vi "Save_Time_Traces_low.vi"(0 "Data Type":T1, 1 "Full Header Info?":bool, 2 "Put each block into separate file":bool, 3 "Precision":i16=2, 5 "No of desired samples/ch":i32, 7 "Data to save":i32[](array[ring])=[1] items=["LDA (V)", "LDA (U)", "Save Nothing"], 9 "File Extension":string=".xls", 11 "Down Sample":i32=1, 12 "Leave space between blocks?":bool, 13 "Time Series":enum16{"Milliseconds", "Seconds"}(ring), 14 "Separation Character":string="\t") -> ()   [LabVIEW 2011]
uses:
  Controls/Instrument_Array.ctl
  Globals/Meas_global.vi
  Acquisition/PWA/PWAtasksGLOBAL.vi
  Globals/Plug_in_data_global.vi
  Globals/LDA_meas_global_1.vi
panel:
  # "Run this VI to update the channel names"
  # "0 means disabled"
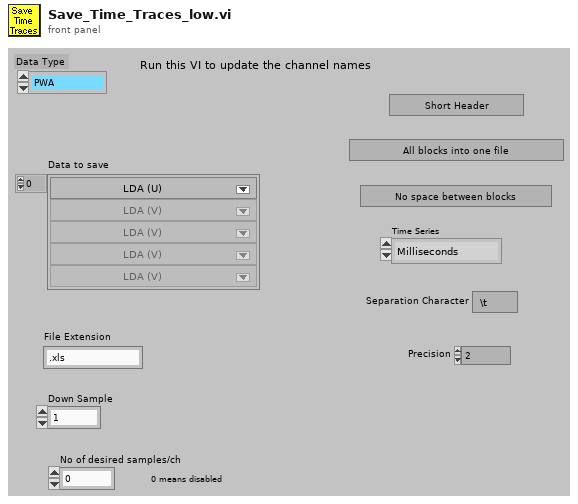
[diagram p1: front panel]
types:
  T1 = typedef "Instrument_Array.ctl" = enum16{"PWA", "LDA", "Analogue"}
  T2 = typedef "Analysis_info_cluster.ctl" = cluster{"Colour":u32, "Inst type":T3, "Inst name":string, "Symbol":string, "Code name":string, "Extra Info":string, "Inst Array":T1, "Index":i32, "Voltage Index":i32, "Extra Titles":string[], "Extra Values":string[]}
  T3 = typedef "Inst_type.ctl" = enum16{"Propeller anemometer", "Raw voltage", "Pressure Transducer", "Pitot-static tube", "Preston tube", "Hot wire", "Cross wire 1", "Cross wire 2", "Generic Linear", "Generic Polynomial", "Generic BackPoly", "Fast FID", "Thermocouple", "Cold wire", "Pulsed Wire", "LDA Vel", "LDA Tran time", "LDA Arr time"}
  T4 = typedef "Trigger_Mode.ctl" = enum16{"Free Running", "Start on Trigger", "Trigger Every Block", "Trigger Every Sample"}
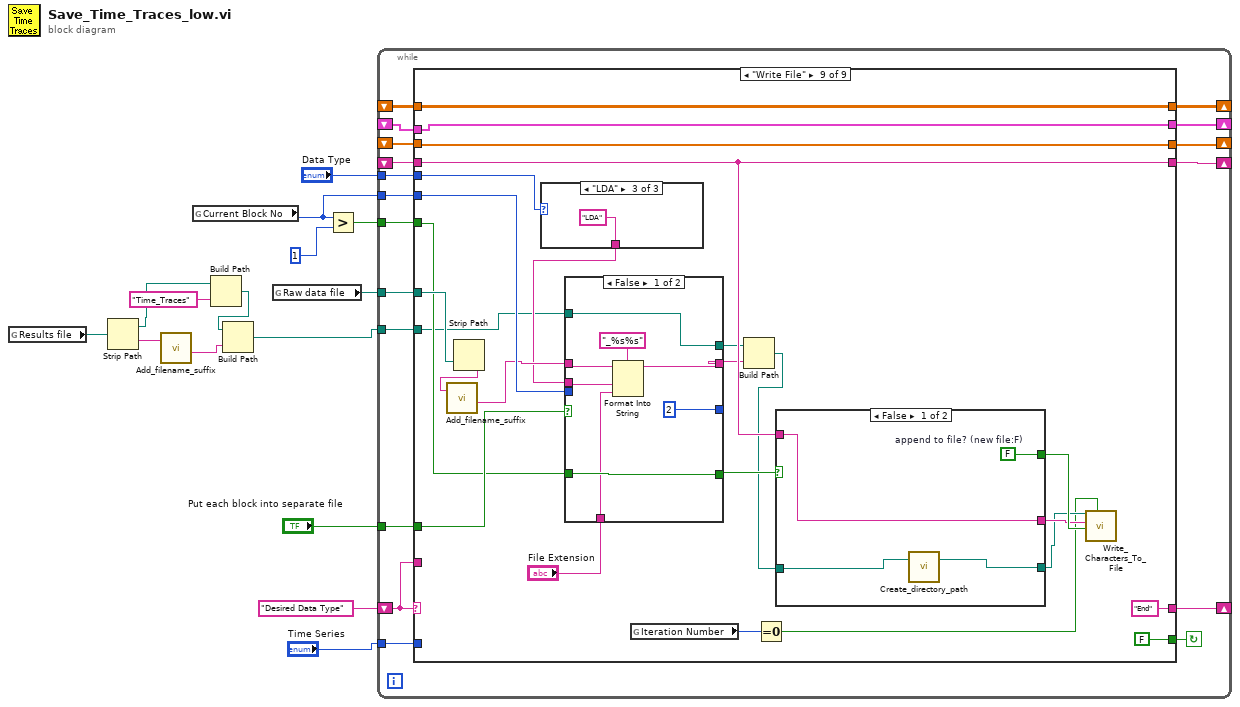
[diagram p0: block diagram]
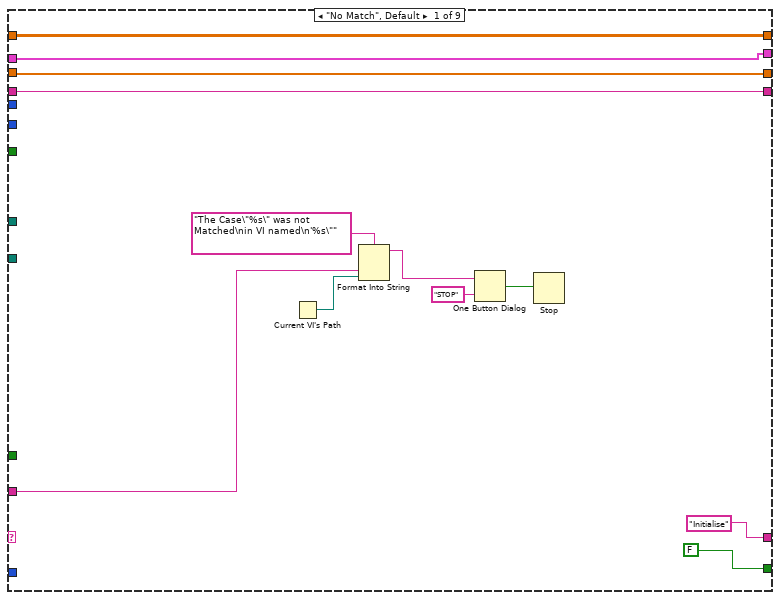
[diagram p2: hidden frame]
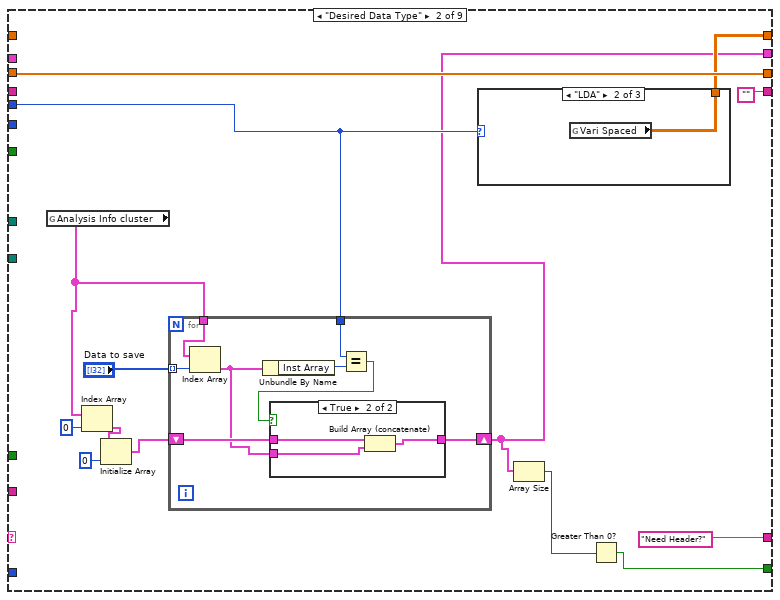
[diagram p3: hidden frame]
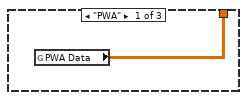
[diagram p5: hidden frame]
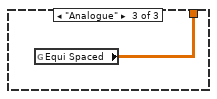
[diagram p6: hidden frame]
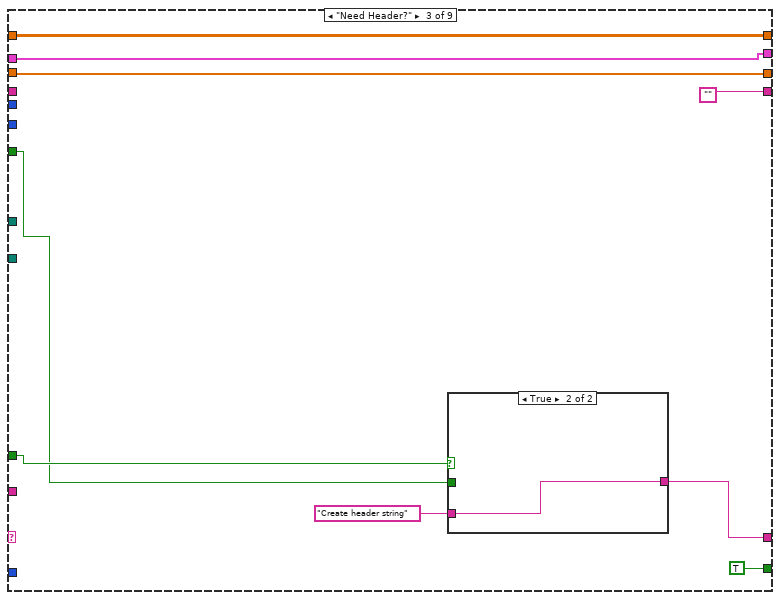
[diagram p7: hidden frame]
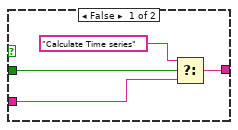
[diagram p8: hidden frame]
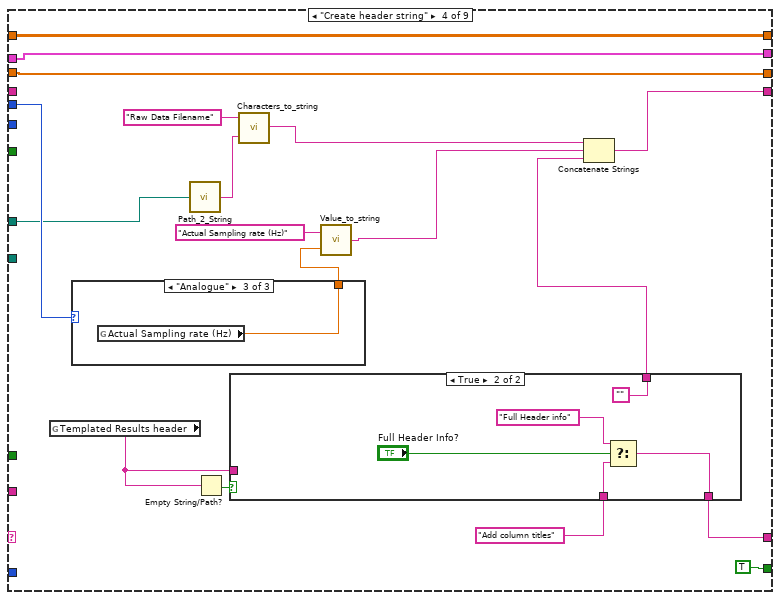
[diagram p9: hidden frame]
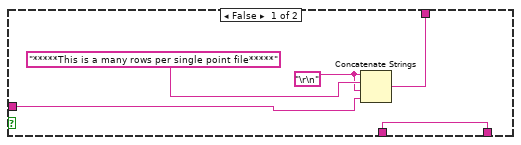
[diagram p10: hidden frame]
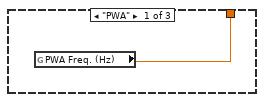
[diagram p11: hidden frame]
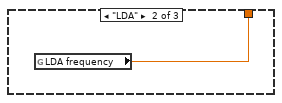
[diagram p12: hidden frame]
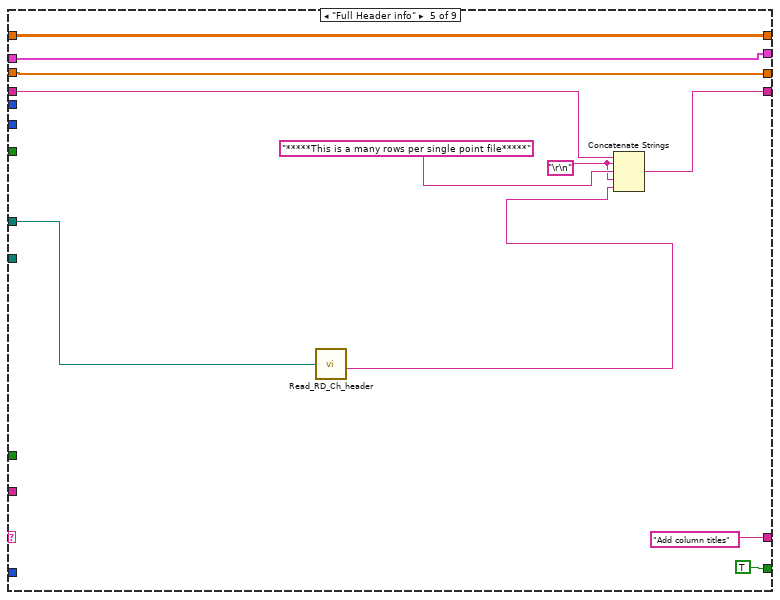
[diagram p13: hidden frame]
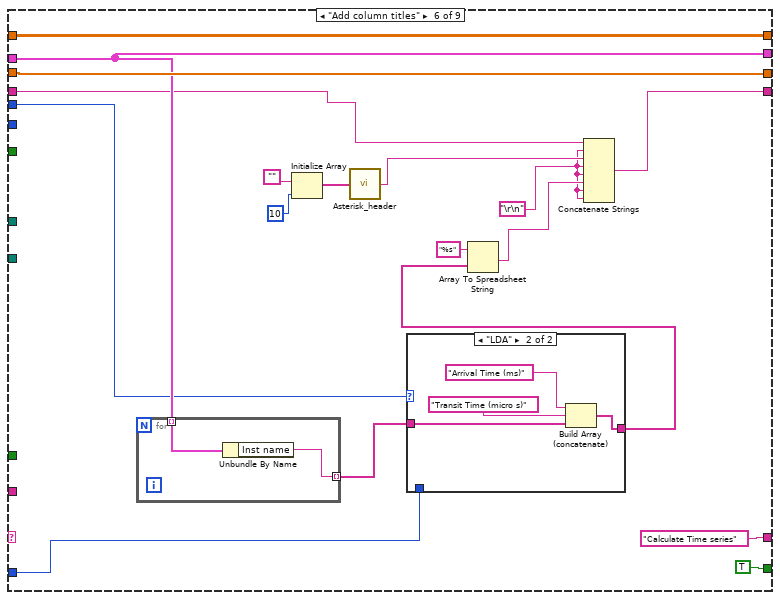
[diagram p14: hidden frame]
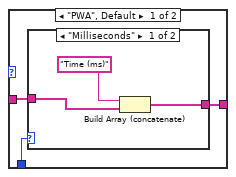
[diagram p15: hidden frame]
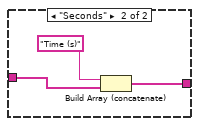
[diagram p16: hidden frame]
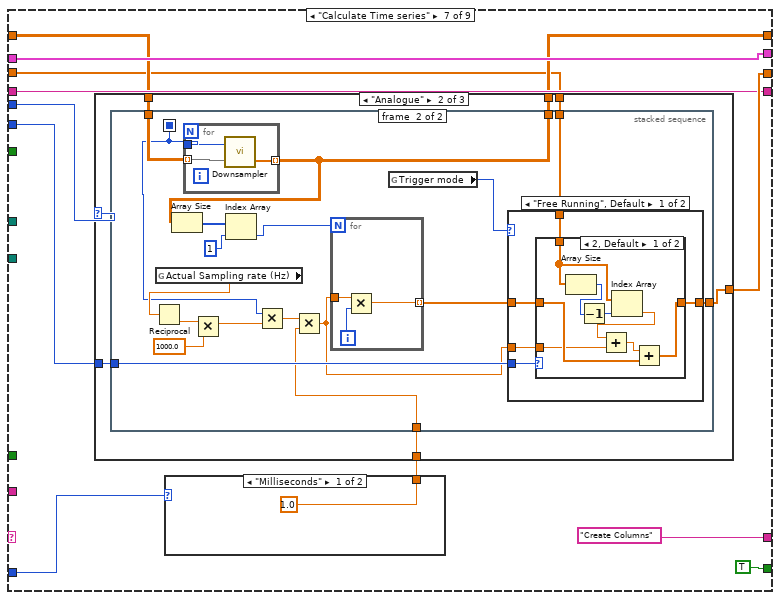
[diagram p17: hidden frame]
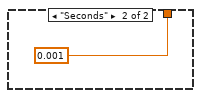
[diagram p18: hidden frame]
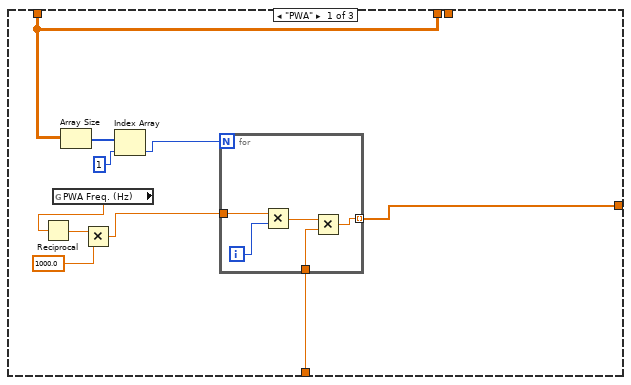
[diagram p19: hidden frame]
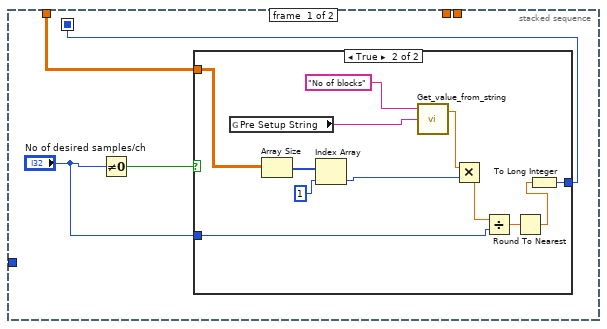
[diagram p20: hidden frame]
diagram:
  n1 = global read "Meas_global.vi" "Results file"() -> (w7:path)
  n2 = Strip Path(path=w7) -> (stripped path=w3:path, name=w6:string)
  n3 = call "Add_filename_suffix.vi"("Filename"=w6) -> ("Base name"=w5:string)  [unwired: 1 in, 3 out]
  n4 = global read "Meas_global.vi" "Current Block No"() -> (w11:i32)
  n5 = Build Path(base path=w3, name or relative path="Time_Traces") -> (appended path=w1:path)
  n6 = Build Path(base path=w1, name or relative path=w5) -> (appended path=w4:path)
  n7 = global read "Meas_global.vi" "Raw data file"() -> (w8:path)
  n8 = Greater?(x=w11, y=1) -> (0:w12:bool)
  n9 = while {
    shift-left: "Desired Data Type" -> [w31]
    shift-right: [w32] -> _
    shift-right: [w28] -> _
    shift-left: _ -> [w27]
    tunnel: "Put each block into separate file" -> [w30]
    tunnel: w8 -> [w29]
    tunnel: w12 -> [w26]
    shift-right: [w25] -> _
    shift-left: _ -> [w24]
    tunnel: w11 -> [w23]
    shift-right: [w22] -> _
    shift-left: _ -> [w21]
    tunnel: "Time Series" -> [w20]
    tunnel: "Data Type" -> [w19]
    shift-right: [w18] -> _
    shift-left: _ -> [w17]
    tunnel: w4 -> [w16]
    stop <- w33 continue-if-true
    n10 = case shown="\"Write File\"" w31 {
      tunnel: [FALSE w47 TRUE TRUE TRUE TRUE TRUE TRUE FALSE] -> w33
      tunnel: ["Initialise" "Need Header?" w80 w90 "Add column titles" ("t") "Calculate Time series" ("t") "Create Columns" ("t") "Write File" "End" ("t")] -> w32
      tunnel: w31 -> [w40 _ _ _ _ _ _ _ _]
      tunnel: w30 -> [_ _ w79 _ _ _ _ _ w346]
      tunnel: w29 -> [_ _ _ w95 w121 _ _ _ w356]
      tunnel: [w37 "" "" w103 w122 w146 w172 w273 w352] -> w28
      tunnel: w27 -> [w37 _ _ _ w123 w137 w172 w275 w352]
      tunnel: w26 -> [_ _ w78 _ _ _ _ _ w342]
      tunnel: [w36 w58 w82 w102 w129 w144 w174 w267 w349] -> w25
      tunnel: w24 -> [w36 w58 w82 w102 w129 w144 w165 w267 w349]
      tunnel: w23 -> [_ _ _ _ _ _ w164 _ w348]
      tunnel: [w35 w57 w75 w99 w128 w142 w166 w271 w343] -> w22
      tunnel: w21 -> [w35 _ w75 w99 w128 w142 w167 w271 w343]
      tunnel: w20 -> [_ _ _ _ _ w131 w171 w270 _]
      tunnel: w19 -> [_ w54 _ w97 _ w134 w169 w266 w338]
      tunnel: [w34 w46 w76 w96 w126 w141 w168 w268 w339] -> w18
      tunnel: w17 -> [w34 _ w76 w96 w126 w141 w168 w268 w339]
      tunnel: w16 -> [_ _ _ _ _ _ _ _ w335]
      frame "No Match", Default {
        n11 = Current VI's Path() -> (path=w39:path)
        n12 = Format Into String(format string="The Case\"%s\" was not Matched\nin VI named\n'%s\"" ("Format String"), w40, w39) -> (resulting string=w43:string)  [unwired: 2 in, 1 out]
        n13 = One Button Dialog(message=w43, button name ("OK")="STOP") -> (true=w41:bool)
        n14 = Stop(stop? (T)=w41) -> ()
      }
      frame "Desired Data Type" {
        n15 = global read "Meas_global.vi" "Analysis Info cluster"() -> (w50:T2[])
        n16 = Index Array(array=w50, index=0) -> (element=w51:T2)
        n17 = Initialize Array(w51, 0 ("dimension size")) -> (w53:T2[])
        n18 = for {
          tunnel: w50 -> [w67]
          tunnel: "Data to save" -> [w66] mode=indexing
          tunnel: w54 -> [w64]
          shift-right: [w60] -> w46
          shift-left: w53 -> [w62]
          n19 = Index Array(array=w67, index=w66) -> (element=w61:T2)
          n20 = Unbundle By Name(w61) -> ("Inst Array"=w65:T1)
          n21 = Equal?(x=w64, y=w65) -> (x = y?=w63:bool)
          n22 = case shown="True" w63 {
            tunnel: w62 -> [w68 w71]
            tunnel: w61 -> [_ w70]
            tunnel: [w68 w69] -> w60
            frame False {
            }
            frame True {
              n23 = Build Array (concatenate)(w71, w70) -> (w69:T2[])
            }
          }
        }
        n24 = case shown="\"LDA\"" w54 {
          tunnel: [w72 w73 w74] -> w57
          frame "PWA" {
            n25 = global read "PWAtasksGLOBAL.vi" "PWA Data"() -> (w72:dbl[][])
          }
          frame "LDA" {
            n26 = global read "Plug_in_data_global.vi" "Vari Spaced"() -> (w73:dbl[][])
          }
          frame "Analogue" {
            n27 = global read "Plug_in_data_global.vi" "Equi Spaced"() -> (w74:dbl[][])
          }
        }
        n28 = Array Size(array=w46) -> (size(s)=w48:i32)
        n29 = Greater Than 0?(x=w48) -> (x > 0?=w47:bool)
      }
      frame "Need Header?" {
        n30 = case shown="True" w79 {
          tunnel: [w87 w88] -> w80
          tunnel: w78 -> [w86 _]
          tunnel: "Create header string" -> [w84 w88]
          frame False {
            n31 = Select(t="Calculate Time series", s=w86, f=w84) -> (s? t:f=w87:string)
          }
          frame True {
          }
        }
      }
      frame "Create header string" {
        n32 = global read "Plug_in_data_global.vi" "Templated Results header"() -> (w92:string)
        n33 = case shown="\"Analogue\"" w97 {
          tunnel: [w117 w118 w119] -> w98
          frame "PWA" {
            n34 = global read "PWAtasksGLOBAL.vi" "PWA Freq. (Hz)"() -> (w117:dbl)
          }
          frame "LDA" {
            n35 = global read "Meas_global.vi" "LDA frequency"() -> (w118:dbl)
          }
          frame "Analogue" {
            n36 = global read "Meas_global.vi" "Actual Sampling rate (Hz)"() -> (w119:dbl)
          }
        }
        n37 = call "Path_2_String.vi"("Real Path"=w95) -> ("Path String"=w94:string)
        n38 = Empty String/Path?(string/path=w92) -> (empty?=w93:bool)
        n39 = case shown="True" w93 {
          tunnel: w92 -> [w109 _]
          tunnel: "Add column titles" ("t") -> [w108 w114]
          tunnel: [w108 w113] -> w90
          tunnel: [w107 ""] -> w89
          frame False {
            w110 = "\r\n"
            n40 = Concatenate Strings(w110, "*****This is a many rows per single point file*****", w110, w109) -> (w107:string)
          }
          frame True {
            n41 = Select(t="Full Header info", s="Full Header Info?", f=w114) -> (s? t:f=w113:string)
          }
        }
        n42 = call "Characters_to_string.vi"("Characters to write"=w94, "Label for characters"="Raw Data Filename") -> ("Output string"=w105:string)
        n43 = call "Value_to_string.vi"("Value"=w98, "Label for value"="Actual Sampling rate (Hz)") -> ("Output string"=w100:string)  [unwired: 1 in]
        n44 = Concatenate Strings(w105, w100, w89) -> (w103:string)
      }
      frame "Full Header info" {
        w124 = "\r\n"
        n45 = call "Read_RD_Ch_header.vi"("Raw data file"=w121) -> ("Ch string"=w120:string)  [unwired: 3 out]
        n46 = Concatenate Strings(w123, w124, "*****This is a many rows per single point file*****", w124, w120) -> (w122:string)
      }
      frame "Add column titles" {
        w135 = "\r\n"
        n47 = for {
          tunnel: [w162] -> w133 mode=indexing
          tunnel: w141 -> [w163] mode=indexing
          n48 = Unbundle By Name(w163) -> ("Inst name"=w162:string)
        }
        n49 = Initialize Array("", 10) -> (w138:string[])
        n50 = call "Asterisk_header.vi"("Channel names"=w138) -> ("Header string"=w136:string)
        n51 = case shown="\"LDA\"" w134 {
          tunnel: w133 -> [w151 w159]
          tunnel: [w150 w158] -> w132
          tunnel: w131 -> [w149 _]
          frame "PWA", Default {
            n52 = case shown="\"Milliseconds\"" w149 {
              tunnel: w151 -> [w154 w157]
              tunnel: [w153 w156] -> w150
              frame "Milliseconds" {
                n53 = Build Array (concatenate)("Time (ms)", w154) -> (w153:string[])
              }
              frame "Seconds" {
                n54 = Build Array (concatenate)("Time (s)", w157) -> (w156:string[])
              }
            }
          }
          frame "LDA" {
            n55 = Build Array (concatenate)("Arrival Time (ms)", "Transit Time (micro s)", w159) -> (w158:string[])
          }
        }
        n56 = Array To Spreadsheet String(array=w132, 3:"%s" ("format string")) -> (spreadsheet string=w143:string)  [unwired: 1 out]
        n57 = Concatenate Strings(w137, w135, w136, w135, w135, w143, w135, w135) -> (w146:string)
      }
      frame "Calculate Time series" {
        n58 = case shown="\"Milliseconds\"" w171 {
          tunnel: [1.0 0.001] -> w170
          frame "Milliseconds" {
          }
          frame "Seconds" {
          }
        }
        n59 = case shown="\"Analogue\"" w169 {
          tunnel: [w179 w195 w256] -> w174
          tunnel: w170 -> [w181 w198 w257]
          tunnel: w167 -> [w178 w197 w255]
          tunnel: [w178 w196 w255] -> w166
          tunnel: w165 -> [_ w194 _]
          tunnel: w164 -> [_ w193 _]
          frame "PWA" {
            n60 = global read "PWAtasksGLOBAL.vi" "PWA Freq. (Hz)"() -> (w180:dbl)
            n61 = Reciprocal(x=w180) -> (1/x=w187:dbl)
            n62 = Array Size(array=w178) -> (size(s)=w184:i32[])
            n63 = Multiply(x=w187, y=1000.0) -> (x*y=w185:dbl)
            n64 = Index Array(array=w184, index=1) -> (element=w182:i32)
            n65 = for {
              N: w182 -> [_]
              tunnel: w185 -> [w191]
              tunnel: [w189] -> w179 mode=indexing
              tunnel: w181 -> [w188]
              i -> [w192]
              n66 = Multiply(x=w191, y=w192) -> (x*y=w190:dbl)
              n67 = Multiply(x=w190, y=w188) -> (x*y=w189:dbl)
            }
          }
          frame "Analogue" {
            n68 = stacked-sequence {
              seq-local: [w200 _] -> [_ w220]
              tunnel: w198 -> [_ w217]
              tunnel: w197 -> [w202 w227]
              tunnel: [_ w225] -> w196
              tunnel: [_ w223] -> w195
              tunnel: w194 -> [_ w221]
              tunnel: w193 -> [_ w219]
              frame #0 {
                n69 = Not Equal To 0?(x="No of desired samples/ch") -> (x != 0?=w199:bool)
                n70 = case shown="True" w199 {
                  tunnel: w202 -> [_ w211]
                  tunnel: "No of desired samples/ch" -> [_ w207]
                  tunnel: ["Down Sample" w204] -> w200
                  frame False {
                  }
                  frame True {
                    n71 = global read "Meas_global.vi" "Pre Setup String"() -> (w214:string)
                    n72 = Array Size(array=w211) -> (size(s)=w213:i32[])
                    n73 = Index Array(array=w213, index=1) -> (element=w209:i32)
                    n74 = call "Get_value_from_string.vi"("Input string"=w214, "Variable name"="No of blocks") -> ("Value"=w210:dbl)  [unwired: 1 in, 1 out]
                    n75 = Multiply(x=w210, y=w209) -> (x*y=w208:dbl)
                    n76 = Divide(x=w208, y=w207) -> (x/y=w206:dbl)
                    n77 = Round To Nearest(number=w206) -> (nearest integer value=w205:dbl)
                    n78 = To Long Integer(number=w205) -> (32bit integer=w204:i32)
                  }
                }
              }
              frame #1 {
                n79 = global read "Meas_global.vi" "Actual Sampling rate (Hz)"() -> (w228:dbl)
                n80 = Reciprocal(x=w228) -> (1/x=w233:dbl)
                n81 = for {
                  tunnel: w227 -> [w251] mode=indexing
                  tunnel: w220 -> [w250]
                  tunnel: [w249] -> w225 mode=indexing
                  n82 = call "Downsampler.vi"("Input Array"=w251, "Averaging samples"=w250) -> ("Downsampled Array"=w249:dbl[])  [unwired: 1 out]
                }
                n83 = Array Size(array=w225) -> (size(s)=w231:i32[])
                n84 = Multiply(x=w233, y=1000.0) -> (x*y=w226:dbl)
                n85 = Index Array(array=w231, index=1) -> (element=w229:i32)
                n86 = Multiply(x=w220, y=w226) -> (x*y=w218:dbl)
                n87 = Multiply(x=w218, y=w217) -> (x*y=w216:dbl)
                n88 = for {
                  N: w229 -> [_]
                  tunnel: w216 -> [w253]
                  tunnel: [w252] -> w222 mode=indexing
                  i -> [w254]
                  n89 = Multiply(x=w253, y=w254) -> (x*y=w252:dbl)
                }
                n90 = global read "Meas_global.vi" "Trigger mode"() -> (w224:T4)
                n91 = case shown="\"Free Running\", Default" w224 {
                  tunnel: w219 -> [w238 _]
                  tunnel: [w237 w248] -> w223
                  tunnel: w222 -> [w236 w248]
                  tunnel: w221 -> [w235 _]
                  tunnel: w216 -> [w234 _]
                  frame "Free Running", Default {
                    n92 = case shown="2, Default" w238 {
                      tunnel: [w242 w247] -> w237
                      tunnel: w236 -> [w243 w247]
                      tunnel: w235 -> [w244 _]
                      tunnel: w234 -> [w239 _]
                      frame 2, Default {
                        n93 = Array Size(array=w244) -> (size(s)=w245:i32)
                        n94 = Decrement(x=w245) -> (x-1=w246:i32)
                        n95 = Index Array(array=w244, index=w246) -> (element=w240:dbl)
                        n96 = Add(x=w240, y=w239) -> (x+y=w241:dbl)
                        n97 = Add(x=w241, y=w243) -> (x+y=w242:dbl[])
                      }
                      frame 1 {
                      }
                    }
                  }
                  frame "Trigger Every Block" {
                  }
                }
              }
            }
          }
          frame "LDA" {
            n98 = global read "LDA_meas_global_1.vi" "Arrival times"() -> (w259:dbl[])
            n99 = for {
              shift-right: [w262] -> _
              shift-left: 0.0 -> [w264]
              tunnel: w259 -> [w263] mode=indexing
              tunnel: [w261] -> w256 mode=indexing
              tunnel: w257 -> [w260]
              n100 = Add(x=w264, y=w263) -> (x+y=w262:dbl)
              n101 = Multiply(x=w262, y=w260) -> (x*y=w261:dbl)
            }
          }
        }
      }
      frame "Create Columns" {
        n102 = Array Size(array=w268) -> (size(s)=w278:i32)
        n103 = Decrement(x=w278) -> (x-1=w279:i32)
        n104 = global read "LDA_meas_global_1.vi" "Transit times"() -> (w265:dbl[])
        n105 = for {
          shift-right: [w296] -> w274
          shift-left: "" -> [w291]
          tunnel: "Separation Character" -> [w282]
          tunnel: w268 -> [w286]
          tunnel: w271 -> [w294]
          tunnel: w279 -> [w290]
          tunnel: w267 -> [w288] mode=indexing
          tunnel: w270 -> [w287]
          tunnel: w266 -> [w285]
          tunnel: w265 -> [w284]
          i -> [w283]
          n106 = case shown="\"Milliseconds\"" w287 {
            tunnel: [w308 w312] -> w281
            tunnel: w282 -> [w307 w311]
            tunnel: w288 -> [w306 w310]
            frame "Seconds" {
              n107 = Format Into String(format string="%.4f%s", w306, w307) -> (resulting string=w308:string)  [unwired: 2 in, 1 out]
            }
            frame "Milliseconds" {
              n108 = Format Into String(format string="%.2f%s", w310, w311) -> (resulting string=w312:string)  [unwired: 2 in, 1 out]
            }
          }
          n109 = Index Array(array=w294, index (col)=w283) -> (element=w293:dbl[])  [unwired: 1 in]
          n110 = case shown="\"LDA\"" w285 {
            tunnel: w284 -> [_ w304]
            tunnel: w283 -> [_ w303]
            tunnel: w282 -> [_ w300]
            tunnel: [w297 w299] -> w280
            tunnel: w281 -> [w297 w298]
            frame "PWA", Default {
            }
            frame "LDA" {
              n111 = Index Array(array=w304, index=w303) -> (element=w301:dbl)
              n112 = Format Into String(format string="%.2f%s", initial string=w298, w301, w300) -> (resulting string=w299:string)  [unwired: 1 in, 1 out]
            }
          }
          n113 = for {
            shift-right: [w322] -> w292
            shift-left: w280 -> [w324]
            tunnel: w282 -> [w321]
            tunnel: w293 -> [w320]
            tunnel: w290 -> [w317]
            tunnel: "Precision" -> [w315]
            tunnel: w286 -> [w314] mode=indexing
            i -> [w318]
            n114 = Unbundle By Name(w314) -> ("Index"=w313:i32)
            n115 = Index Array(array=w320, index=w313) -> (element=w319:dbl)
            n116 = Equal?(x=w318, y=w317) -> (x = y?=w316:bool)
            n117 = Number To Fractional String(number=w319, precision (6)=w315) -> (F-format string=w323:string)  [unwired: 2 out]
            n118 = case shown="True" w316 {
              tunnel: w324 -> [w328 w331]
              tunnel: w323 -> [w327 w330]
              tunnel: [w326 w329] -> w322
              tunnel: w321 -> [w325 _]
              frame False {
                n119 = Concatenate Strings(w328, w327, w325) -> (w326:string)
              }
              frame True {
                n120 = Concatenate Strings(w331, w330) -> (w329:string)
              }
            }
          }
          n121 = Concatenate Strings(w291, w292, "\r\n") -> (w296:string)
        }
        n122 = Concatenate Strings(w275, w274) -> (w273:string)
      }
      frame "Write File" {
        n123 = Strip Path(path=w356) -> (name=w340:string)  [unwired: 1 out]
        n124 = call "Add_filename_suffix.vi"("Filename"=w340) -> ("Base name"=w341:string)  [unwired: 1 in, 3 out]
        n125 = case shown="\"LDA\"" w338 {
          tunnel: ["PWA" "AN" "LDA"] -> w337
          frame "PWA" {
          }
          frame "Analogue" {
          }
          frame "LDA" {
          }
        }
        n126 = case shown="False" w346 {
          tunnel: w341 -> [w362 w373]
          tunnel: w348 -> [_ w370]
          tunnel: [w361 w376] -> w347
          tunnel: w342 -> [w367 _]
          tunnel: [w367 FALSE] -> w345
          tunnel: [w366 w372] -> w344
          tunnel: w335 -> [w366 w374]
          tunnel: [2 ("y") 3 ("y")] -> _
          tunnel: w337 -> [w363 w369]
          tunnel: "File Extension" -> [w360 w368]
          frame False {
            n127 = Format Into String(format string="_%s%s", initial string=w362, w363, w360) -> (resulting string=w361:string)  [unwired: 1 in, 1 out]
          }
          frame True {
            n128 = Format Into String(format string="_%s_%d%s", initial string=w373, w369, w370, w368) -> (resulting string=w376:string)  [unwired: 1 in, 1 out]
            n129 = Build Path(base path=w374, name or relative path=w373) -> (appended path=w372:path)
          }
        }
        n130 = global read "Meas_global.vi" "Iteration Number"() -> (w333:i32)
        n131 = Build Path(base path=w344, name or relative path=w347) -> (appended path=w334:path)
        n132 = Equal To 0?(x=w333) -> (x = 0?=w332:bool)
        n133 = case shown="False" w345 {
          tunnel: [w378 w386] -> w354
          tunnel: w352 -> [w378 w385]
          tunnel: [w381 w384] -> w355
          tunnel: w334 -> [w380 w382]
          tunnel: [w379 w382] -> w353
          frame False {
            w381 = FALSE  # append to file? (new file:F)
            n134 = call "Create_directory_path.vi"("Path name"=w380) -> ("Path name Out"=w379:path)  [unwired: 1 in, 1 out]
          }
          frame True {
            w384 = TRUE  # append to file? (new file:F)
            n135 = case shown="True" "Leave space between blocks?" {
              tunnel: [w387 w390] -> w386
              tunnel: w385 -> [w387 w389]
              frame False {
              }
              frame True {
                n136 = Concatenate Strings("\r\n", w389) -> (w390:string)
              }
            }
          }
        }
        n137 = call "Write_Characters_To_File.vi"("file path (dialog if empty)"=w353, "advisory dialog? (display:T)"=w332, "character string"=w354, "append to file? (new file:F)"=w355) -> ()  [unwired: 1 in, 4 out]
      }
    }
  }
